vi "Benchmark Project.vi"() -> ()   [LabVIEW 2017]
doc: "This example gathers timing information about a VI's execution by running the VI over several iterations. The example obtains several consecutive timestamps, which are stored in an array and used to produce a histogram of execution time. The example can self-calibrate by subtracting out the overhead of calling NI Get Timestamp.vi from the array of timing data."
uses:
  <vilib>/rvi/errors/niLvFpgaAdjustHostInterfaceError.vi
  <vilib>/Utility/error.llb/Error Cluster From Error Code.vi
  <vilib>/nisyscfg/Close (System).vi
  Globals/Global - All RT Loop Stop.vi
  <vilib>/rvi/interface/nirviReadWriteControl/nirviReadWriteControl.xnode
  <vilib>/NI_Real-Time Target Support.lvlib
  UI Error Handlers/support/Message Queue/Message Queue.lvlib
  NiFpgaLv.dll
  <vilib>/rvi/interface/Simulation/niFpgaSimulationCallBeginRW.vi
  <vilib>/nisyscfg/nisyscfg.lvlib
panel:
  out "Mean time (us)":dbl format="%.3g"
  out "Max jitter (us)":dbl format="%.3g"
  out "Standard deviation (us)":dbl format="%.3g"
  in  "Warmup iterations":i32=10
  in  "Calibrate?":bool
  in  "Iterations":i32=1000
  out "Execution histogram":T1(graph)
  out "Execution times (us)":dbl[](graph)
  # "Overview: Gathers timing information on VI execution by running it over several iterations.\nRequirements: LabVIEW Real-Time Module\nInstructions:\n1. In Measurement & Automation Explorer, ensure that LabVIEW Real-Time is installed on your RT target.  \n2. From the Project Explorer window, set the IP address of your RT target.\n3. From the front panel, select the number of iterations to run and the number of warmup iterations to exclude from the benchmark.\n4. Enable Calibrate? if you want to exclude the overhead of the timestamping operation.\n5. Open the block diagram and insert the code you want to benchmark in the #CodeNeeded section.\n6. Run the VI."
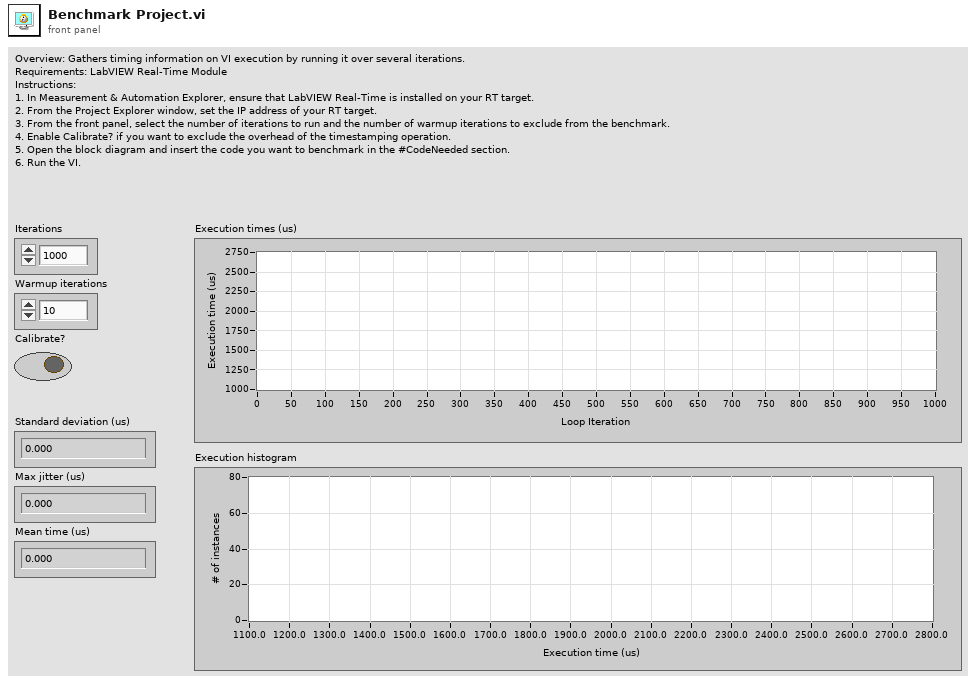
[diagram p1: front panel]
types:
  T1 = cluster{"X Values":dbl[], "Histogram: h(x)":i32[]}
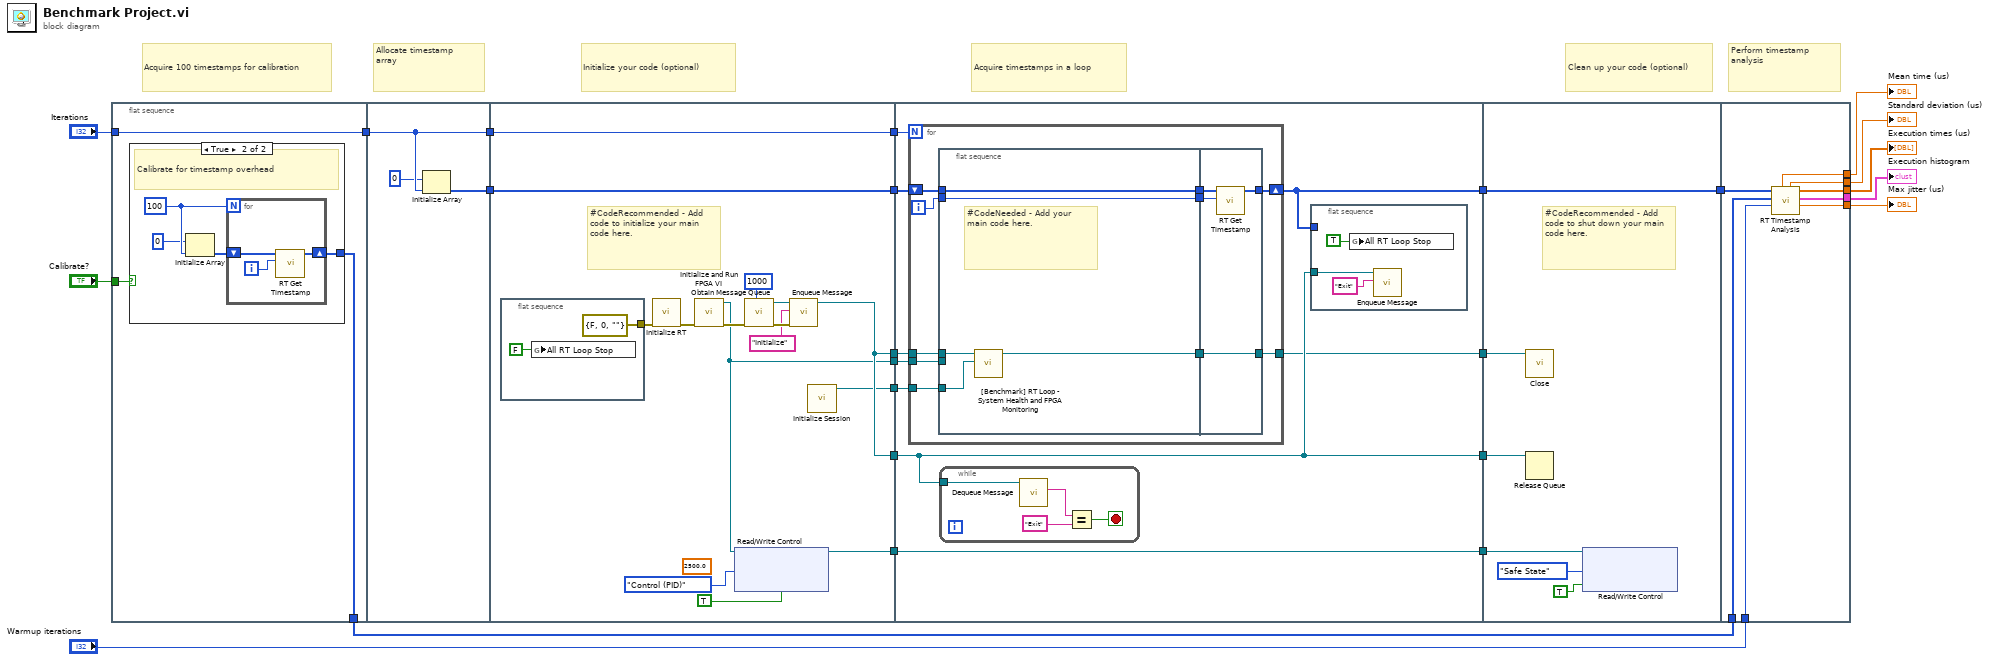
[diagram p0: block diagram]
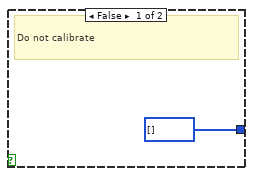
[diagram p2: hidden frame]
diagram:
  # "Perform timestamp analysis"
  # "Clean up your code (optional)"
  # "Acquire timestamps in a loop"
  # "Initialize your code (optional)"
  # "Allocate timestamp array"
  # "Acquire 100 timestamps for calibration"
  n1 = flat-sequence {
    tunnel: "Iterations" -> [w27]
    tunnel: [w27] -> w18
    tunnel: "Calibrate?" -> [w26]
    tunnel: [w25] -> w15
    tunnel: [w37] -> w20
    tunnel: [w38] -> w19
    tunnel: w18 -> [w37]
    tunnel: [w53] -> w22
    tunnel: [w52] -> w21
    tunnel: w20 -> [w53]
    tunnel: w19 -> [w52]
    tunnel: [w44] -> w8
    tunnel: [w42] -> w7
    tunnel: [w44] -> w6
    tunnel: [w40] -> w3
    tunnel: [w39] -> w2
    tunnel: [w60] -> w23
    tunnel: w22 -> [w64]
    tunnel: w21 -> [w63]
    tunnel: w8 -> [w62]
    tunnel: w7 -> [w61]
    tunnel: w6 -> [w59]
    tunnel: [w59] -> w5
    tunnel: [w58] -> w4
    tunnel: w3 -> [w58]
    tunnel: w2 -> [w57]
    tunnel: [w56] -> w1
    tunnel: w23 -> [w96]
    tunnel: [w96] -> w16
    tunnel: w5 -> [w93]
    tunnel: w4 -> [w94]
    tunnel: w1 -> [w91]
    tunnel: w16 -> [w104]
    tunnel: w15 -> [w103]
    tunnel: [w102] -> w9
    tunnel: [w101] -> w13
    tunnel: [w100] -> w12
    tunnel: [w99] -> w14
    tunnel: "Warmup iterations" -> [w98]
    tunnel: [w97] -> w10
    frame #0 {
      n2 = case shown="True" w26 {
        tunnel: [u64[] [] w32] -> w25
        frame False {
          # "Do not calibrate"
        }
        frame True {
          w30 = 100
          # "Calibrate for timestamp overhead"
          n3 = Initialize Array(u64 0, w30) -> (w31:u64[])
          n4 = for {
            N: w30 -> [_]
            shift-right: [w33] -> w32
            shift-left: w31 -> [w34]
            i -> [w35]
            n5 = call <vilib>:"RT Get Timestamp.vi"("iteration"=w35, "timestamp array in"=w34) -> ("timestamp array out"=w33:u64[])  [unwired: 1 in, 8 out]
          }
        }
      }
    }
    frame #1 {
      n6 = Initialize Array(u64 0, w37) -> (w38:u64[])
    }
    frame #2 {
      (unwired) sgl 2500.0 ("Fan Speed Setpoint (RPM)")
      # "#CodeRecommended - Add code to initialize your main code here."
      n7 = flat-sequence {
        tunnel: [errorcluster {"status"=FALSE, "code"=0, "source"=""} ("error constant")] -> w51
        frame #0 {
          n8 = global write "Global - All RT Loop Stop.vi" "All RT Loop Stop"(FALSE) -> ()
        }
      }
      n9 = call "Initialize RT.vi"("error in"=w51) -> ("error out"=w50:errorcluster)  [unwired: 8 in, 2 out]
      n10 = call "Initialize and Run FPGA VI.vi"("error in (no error)"=w50) -> ("error out"=w45:errorcluster, "FPGA VI Reference Out"=w42:refnum<k20>)  [unwired: 9 in]
      n11 = xnode "Read/Write Control"("FPGA VI Reference In"=w42, "New FPGA State"=enum16{"Safe State", "Control (PID)"}."Control (PID)", "Change State"=TRUE) -> ("FPGA VI Reference Out"=w40:refnum<k20>)  [unwired: 1 in, 1 out]
      n12 = call "Obtain Message Queue.vi"("max queue size (-1, unlimited)"=1000, "error in (no error)"=w45) -> ("error out"=w49:errorcluster, "Message Queue"=w48:refnum<queue>)  [unwired: 8 in]
      n13 = call "Enqueue Message.vi"("error in (no error)"=w49, "Message"="Initialize", "Message Queue"=w48) -> ("dup Message Queue"=w44:refnum<queue>)  [unwired: 7 in, 1 out]
      n14 = call <vilib>:"Initialize Session.vi"() -> ("Session out"=w39:refnum<k21>)  [unwired: 10 in, 1 out]
    }
    frame #3 {
      n15 = for {
        N: w64 -> [_]
        shift-right: [w81] -> w60
        shift-left: w63 -> [w80]
        tunnel: w62 -> [w76]
        tunnel: w61 -> [w75]
        tunnel: w57 -> [w74]
        tunnel: [w72] -> w56
        i -> [w79]
        n16 = flat-sequence {
          tunnel: w80 -> [w86]
          tunnel: [w86] -> w78
          tunnel: w79 -> [w85]
          tunnel: [w85] -> w77
          tunnel: w76 -> [w84]
          tunnel: w75 -> [_]
          tunnel: w74 -> [w83]
          tunnel: [w82] -> w73
          tunnel: [w90] -> w81
          tunnel: w78 -> [w88]
          tunnel: w77 -> [w89]
          tunnel: [w87] -> w72
          tunnel: w73 -> [w87]
          frame #0 {
            # "#CodeNeeded - Add your main code here."
            n17 = call "[Benchmark] RT Loop - System Health and FPGA Monitoring.vi"("Session in"=w83, "Message Queue"=w84) -> ("Session out"=w82:refnum<k21>)  [unwired: 9 in]
          }
          frame #1 {
            n18 = call <vilib>:"RT Get Timestamp.vi"("iteration"=w89, "timestamp array in"=w88) -> ("timestamp array out"=w90:u64[])  [unwired: 1 in, 8 out]
          }
        }
      }
      n19 = while {
        tunnel: w59 -> [w71]
        stop <- w68 stop-if-true
        n20 = call "Dequeue Message.vi"("Message Queue"=w71) -> ("Message"=w70:string)  [unwired: 7 in, 3 out]
        n21 = Equal?(x=w70, y="Exit") -> (x = y?=w68:bool)
      }
      n22 = flat-sequence {
        tunnel: w60 -> [_]
        tunnel: w59 -> [w66]
        frame #0 {
          n23 = global write "Global - All RT Loop Stop.vi" "All RT Loop Stop"(TRUE) -> ()
          n24 = call "Enqueue Message.vi"("Message"="Exit", "Message Queue"=w66) -> ()  [unwired: 8 in, 2 out]
        }
      }
    }
    frame #4 {
      # "#CodeRecommended - Add code to shut down your main code here."
      n25 = call-poly <vilib>:"Close.vi"("Session in"=w91) -> ()  [unwired: 10 in, 1 out]
      n26 = Release Queue(queue=w93) -> ()  [unwired: 2 in, 3 out]
      n27 = xnode "Read/Write Control"("FPGA VI Reference In"=w94, "New FPGA State"=enum16{"Safe State", "Control (PID)"}."Safe State", "Change State"=TRUE) -> ()  [unwired: 1 in, 2 out]
    }
    frame #5 {
      n28 = call <vilib>:"RT Timestamp Analysis.vi"("warmup iterations"=w98, "calibration array"=w103, "timestamp array"=w104) -> ("max jitter (uS)"=w101:dbl, "execution histogram"=w102:T1, "execution times (uS)"=w99:dbl[], "standard deviation (uS)"=w100:dbl, "mean time (uS)"=w97:dbl)  [unwired: 1 in, 3 out]
    }
  }
  "Execution times (us)" <- w14
  "Max jitter (us)" <- w13
  "Standard deviation (us)" <- w12
  "Execution histogram" <- w9
  "Mean time (us)" <- w10
